vi "RealTimeMain.vi"() -> ()   [LabVIEW 2015]
uses:
  <vilib>/robotics/Starter Kit/2.0/9632 Host Interface/NI_Robotics_Starter Kit Host_9632_2.0.lvclass
  <vilib>/robotics/Starter Kit/Host Interface/NI_Robotics_Starter Kit Host.lvclass
panel:
  out "Gauge":dbl(knob) scale=0.0..1.0
  out "Array 2":u16[][](array[ring])
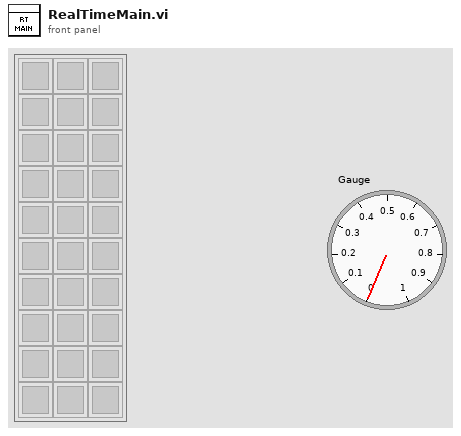
[diagram p1: front panel]
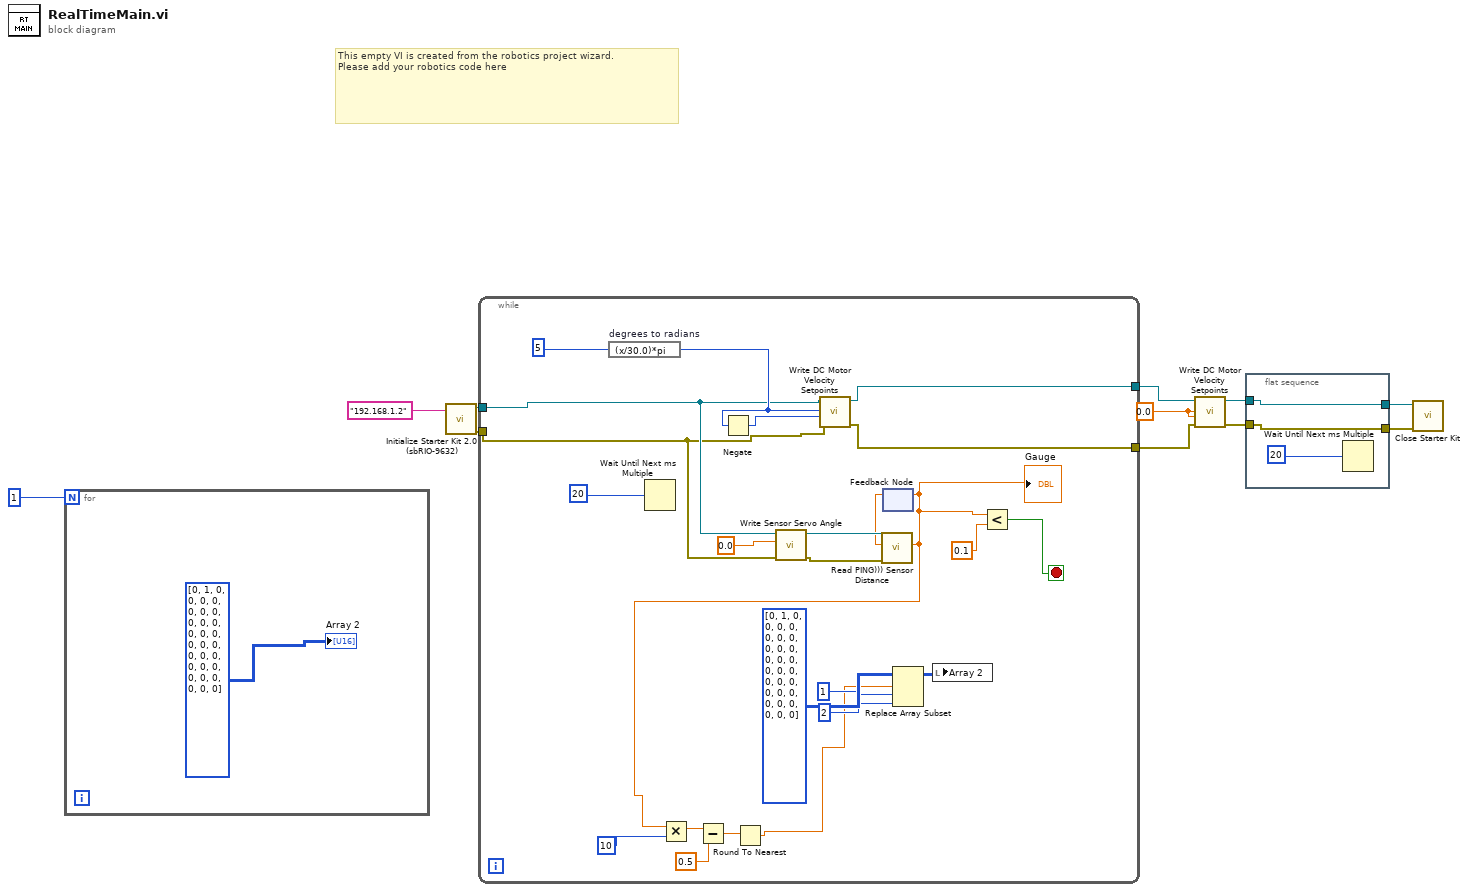
[diagram p0: block diagram]
diagram:
  w8 = 0.0
  # "This empty VI is created from the robotics project wizard.\nPlease add your robotics code here"
  n1 = for {
    N: 1 -> [_]
    "Array 2" <- i32[][] [[0, 1, 0], [0, 0, 0], [0, 0, 0], [0, 0, 0], [0, 0, 0], [0, 0, 0], [0, 0, 0], [0, 0, 0], [0, 0, 0], [0, 0, 0]]
  }
  n2 = call <vilib>:"Initialize Starter Kit 2.0 (sbRIO-9632).vi"("IP address (\"\")"="192.168.1.2") -> ("error out"=w9:errorcluster, "FPGA starter kit host 2.0 out"=w10:refnum<class "NI_Robotics_Starter Kit Host_9632_2.0.lvclass">)  [unwired: 9 in]
  n3 = while {
    tunnel: w10 -> [w30]
    tunnel: w9 -> [w29]
    tunnel: [w35] -> w7
    tunnel: [w34] -> w6
    stop <- w25 stop-if-true
    n4 = expression code="(x/30.0)*pi" "degrees to radians"(5) -> (w33:i32)
    n5 = Wait Until Next ms Multiple(millisecond multiple=20) -> ()  [unwired: 1 out]
    n6 = Negate(x=w33) -> (-x=w32:i32)
    n7 = call <vilib>:"Write Sensor Servo Angle.vi"("error in (no error)"=w29, "ccw servo angle (rad)"=0.0, "starter kit host in"=w30) -> ("error out"=w27:errorcluster, "starter kit host out"=w28:refnum<class "NI_Robotics_Starter Kit Host_9632_2.0.lvclass">)  [unwired: 7 in]
    n8 = call <vilib>:"Write DC Motor Velocity Setpoints.vi"("error in (no error)"=w29, "right motor ccw velocity (rad/s)"=w32, "left motor ccw velocity (rad/s)"=w33, "starter kit host in"=w30) -> ("error out"=w34:errorcluster, "starter kit host out"=w35:refnum<class "NI_Robotics_Starter Kit Host_9632_2.0.lvclass">)  [unwired: 6 in]
    n9 = feedback #1() -> (w26:dbl)  [unwired: 1 in]
    n10 = call <vilib>:"Read PING))) Sensor Distance.vi"("error in (no error)"=w27, "default distance (NaN)"=w26, "starter kit host in"=w28) -> ("distance (m)"=w17:dbl)  [unwired: 5 in, 3 out]
    "Gauge" <- w17
    n11 = Multiply(x=w17, y=10) -> (x*y=w14:dbl)
    n12 = Subtract(x=w14, y=0.5) -> (x-y=w15:dbl)
    n13 = Round To Nearest(number=w15) -> (nearest integer value=w16:dbl)
    n14 = feedback-in #1(w17) -> ()
    n15 = Replace Array Subset(array=i32[][] [[0, 1, 0], [0, 0, 0], [0, 0, 0], [0, 0, 0], [0, 0, 0], [0, 0, 0], [0, 0, 0], [0, 0, 0], [0, 0, 0], [0, 0, 0]], new element=2, index (row)=w16, index (col)=1) -> (w22:i32[][])
    n16 = local write "Array 2"(w22) -> ()
    n17 = Less?(x=w17, y=0.1) -> (x < y?=w25:bool)
  }
  n18 = call <vilib>:"Write DC Motor Velocity Setpoints.vi"("error in (no error)"=w6, "right motor ccw velocity (rad/s)"=w8, "left motor ccw velocity (rad/s)"=w8, "starter kit host in"=w7) -> ("error out"=w2:errorcluster, "starter kit host out"=w3:refnum<class "NI_Robotics_Starter Kit Host_9632_2.0.lvclass">)  [unwired: 6 in]
  n19 = flat-sequence {
    tunnel: [w39] -> w5
    tunnel: [w38] -> w4
    tunnel: w3 -> [w39]
    tunnel: w2 -> [w38]
    frame #0 {
      n20 = Wait Until Next ms Multiple(millisecond multiple=20) -> ()  [unwired: 1 out]
    }
  }
  n21 = call-dynamic "Close Starter Kit.vi"("error in (no error)"=w4, "starter kit host in"=w5) -> ()  [unwired: 9 in, 1 out]
